vi "N-Wave Memory write from DMA - Host.vi"(7 "n":i32=1, 8 "error in":errorcluster, 11 "FPGA VI Reference In":refnum<k20>) -> (0 "FPGA VI Reference Out":refnum<k20>, 3 "error out":errorcluster, 6 "Write memory complete":bool)   [LabVIEW 2014]
uses:
  <vilib>/rvi/interface/common/niFpgaWaitOnOcc.vi
  <vilib>/Utility/error.llb/Error Cluster From Error Code.vi
  <vilib>/rvi/errors/niLvFpgaAdjustHostInterfaceError.vi
  <vilib>/RVI Host/nirviSupport.llb/nirviErrorClusterFromErrorCode.vi
  <vilib>/rvi/interface/nirviMethod/nirviMethod.xnode
  <vilib>/rvi/errors/niLvFpgaMergeErrorWithErrorCode.vi
  <vilib>/rvi/interface/nirviMethod/StockFPGA_InlinedMethodWaitForSingleIRQ.vi
  <vilib>/FPGAPlugInAG/Dynamic/niLvFpga_WaitOnIrq_Dynamic.vi
  <vilib>/FPGAPlugInAG/Dynamic/niLvFpga_AcknowledgeIrq_Dynamic.vi
  <vilib>/FPGAPlugInAG/Dynamic/niLvFpga_ConfigureFifo_Dynamic.vi
  <vilib>/FPGAPlugInAG/Dynamic/niLvFpga_StartFifo_Dynamic.vi
  <vilib>/FPGAPlugInAG/Dynamic/niLvFpga_WriteFifo_Dynamic.vi
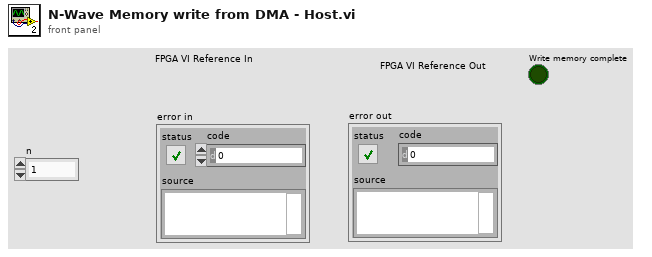
[diagram p1: front panel]
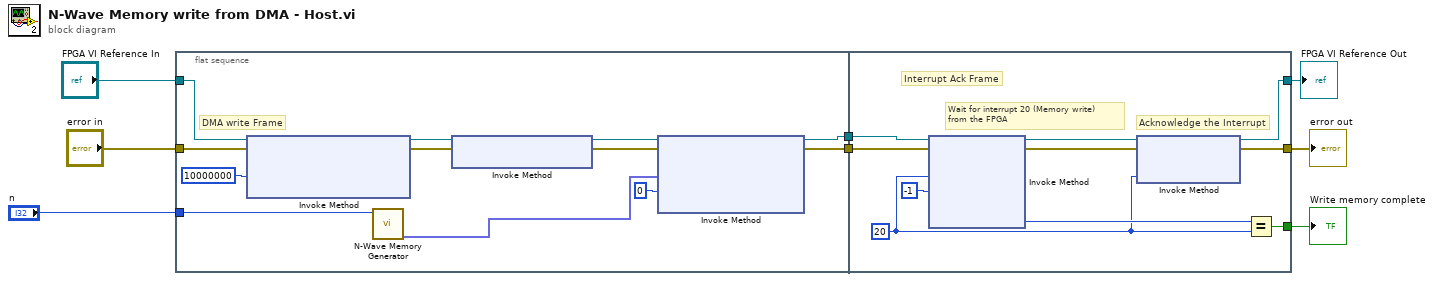
[diagram p0: block diagram]
diagram:
  n1 = flat-sequence {
    tunnel: [w14] -> w8
    tunnel: [w13] -> w7
    tunnel: "error in" -> [w12]
    tunnel: "FPGA VI Reference In" -> [w11]
    tunnel: "n" -> [w9]
    tunnel: [w24] -> w2
    tunnel: [w25] -> w6
    tunnel: w8 -> [w29]
    tunnel: w7 -> [w30]
    tunnel: [w21] -> w5
    frame #0 {
      # "DMA write Frame"
      n2 = xnode "Invoke Method"("FPGA VI Reference In"=w11, "error in"=w12, "Requested Depth"=u32 10000000) -> ("FPGA VI Reference Out"=w19:refnum<k20>, "error out"=w18:errorcluster)  [unwired: 1 out]
      n3 = call "N-Wave Memory Generator.vi"("n"=w9) -> ("FXP Init Data Out"=w10:fxp<+/-,12,12>[])  [unwired: 9 in, 1 out]
      n4 = xnode "Invoke Method"("FPGA VI Reference In"=w19, "error in"=w18) -> ("FPGA VI Reference Out"=w16:refnum<k20>, "error out"=w17:errorcluster)
      n5 = xnode "Invoke Method"("FPGA VI Reference In"=w16, "error in"=w17, "Data"=w10, "Timeout (ms)"=0) -> ("FPGA VI Reference Out"=w14:refnum<k20>, "error out"=w13:errorcluster)  [unwired: 1 out]
    }
    frame #1 {
      w22 = 20 ("IRQ Number(s)")
      # "Acknowledge the Interrupt"
      # "Wait for interrupt 20 (Memory write)\nfrom the FPGA"
      # "Interrupt Ack Frame"
      n6 = xnode "Invoke Method"("FPGA VI Reference In"=w29, "error in"=w30, "IRQ Number(s)"=w22, "Timeout (ms)"=-1) -> ("FPGA VI Reference Out"=w26:refnum<k20>, "error out"=w27:errorcluster, "IRQ(s) Asserted"=w23:i32)  [unwired: 1 out]
      n7 = xnode "Invoke Method"("FPGA VI Reference In"=w26, "error in"=w27, "IRQ Number(s)"=w22) -> ("FPGA VI Reference Out"=w24:refnum<k20>, "error out"=w25:errorcluster)
      n8 = Equal?(x=w23, y=w22) -> (x = y?=w21:bool)
    }
  }
  "error out" <- w6
  "Write memory complete" <- w5
  "FPGA VI Reference Out" <- w2
